vi "KelvinoxRotatorMonitor.vi"() -> ()   [LabVIEW 2019]
uses:
  Utility/Monitor Communication/Kelvinox/Kelvinox_Rotator_Cluster.ctl
  Instrument_Setup.vi
  Equipment/Mercury iXX/Public/Libraries/Auxiliary/Open/Open Auxiliary Device.vi
  Global/Global Variables/Data_Display_global.vi
  Equipment/Mercury iXX/Mercury iXX.lvlib
  Equipment/Mercury iXX/Public/Libraries/Auxiliary.lvlib
panel:
  out "Kelvinox-Rotator-Cluster":T1={"Angle (deg)"=3.4572, "Target Angle (deg)"=3.4572, "Angle SP"=0.0, "Set Angle SP"=FALSE, "Set Angle to Zero"=FALSE} {"Target Angle (deg)" format="%#.2g"; "Angle SP" format="%#.2g"; "Angle (deg)" format="%4.2g"}
  # "Kelvinox Rotator"
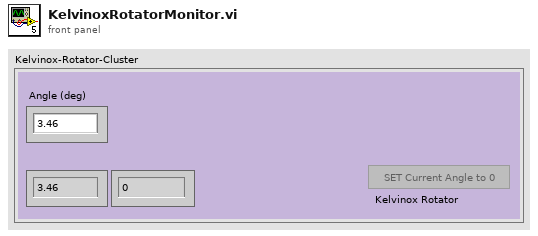
[diagram p1: front panel]
types:
  T1 = typedef "Kelvinox_Rotator_Cluster.ctl" = cluster{"Angle (deg)":dbl, "Target Angle (deg)":dbl, "Angle SP":dbl, "Set Angle SP":bool, "Set Angle to Zero":bool}
  T2 = typedef "Mercury iXX.lvlib/Mercury Reference.ctl" = cluster{"Comms":refnum<visa-resource-name>, "Device ID":string[], "Comms Layer":T3, "Command":string, "Query reference":T4}
  T3 = typedef "Mercury iXX.lvlib/Comms Transport Layer.ctl" = enum16{"Ethernet TCP/IP", "USB", "ISOBus - RS-232", "GPIB"}
  T4 = typedef "Mercury iXX.lvlib/Query Dynamic Reference.ctl" = refnum<vi>
  T5 = typedef "Kelvinox_Rotator_Control.ctl" = cluster{"Angle SP":dbl, "Set Angle SP":bool, "Set Angle to Zero":bool}
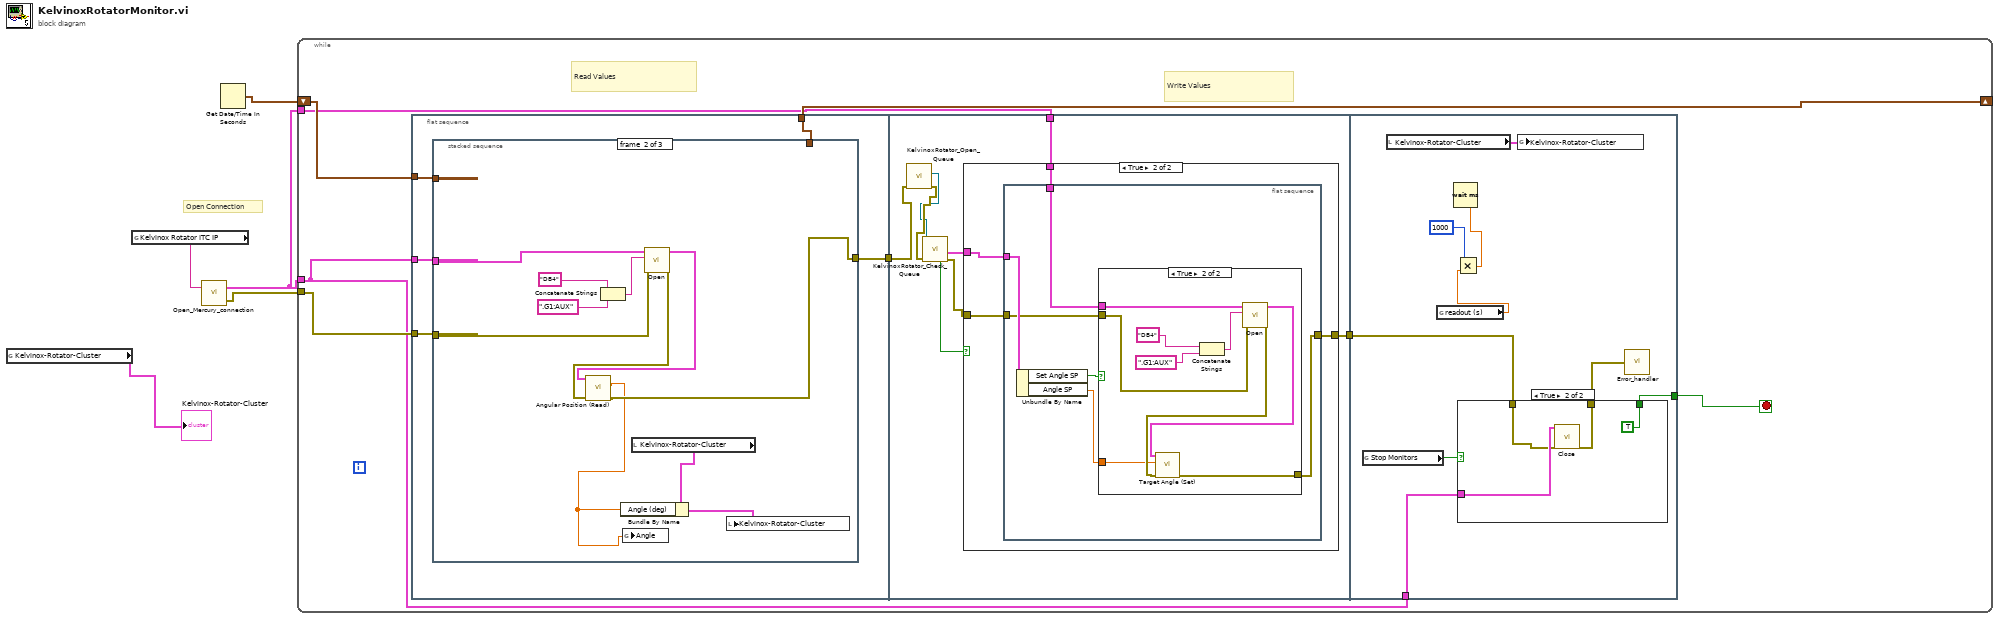
[diagram p0: block diagram]
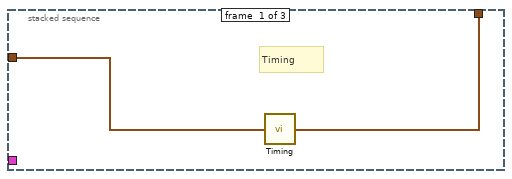
[diagram p2: hidden frame]
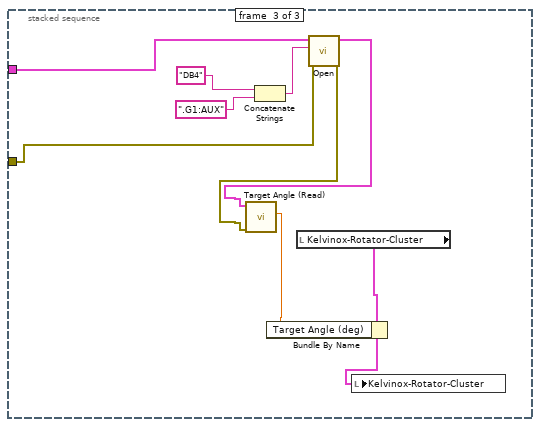
[diagram p3: hidden frame]
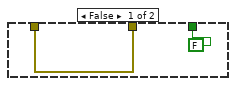
[diagram p6: hidden frame]
diagram:
  # "Open Connection"
  n1 = global read "Data_Display_global.vi" "Kelvinox-Rotator-Cluster"() -> (→"Kelvinox-Rotator-Cluster":T1)
  n2 = global read "Instrument_Setup.vi" "Kelvinox Rotator ITC IP"() -> (w5:string)
  n3 = call "Open_Mercury_connection.vi"("IP Address"=w5) -> ("error out"=w2:errorcluster, "Mercury Reference Out"=w1:T2)  [unwired: 1 in]
  n4 = Get Date/Time In Seconds() -> (seconds since 1Jan1904=w4:timestamp)
  n5 = while {
    tunnel: w1 -> [w7]
    tunnel: w2 -> [w13]
    shift-right: [w11] -> _
    shift-left: w4 -> [w12]
    tunnel: w1 -> [w9]
    stop <- w6 stop-if-true
    # "Write Values"
    # "Read Values"
    n6 = flat-sequence {
      tunnel: w13 -> [w18]
      tunnel: w7 -> [w17]
      tunnel: w12 -> [w16]
      tunnel: [w15] -> w11
      tunnel: [w14] -> w10
      tunnel: w10 -> [w47]
      tunnel: w9 -> [w49]
      tunnel: [w48] -> w8
      tunnel: w8 -> [w73]
      tunnel: w7 -> [w74]
      tunnel: [w72] -> w6
      frame #0 {
        n7 = stacked-sequence {
          tunnel: w17 -> [_ w29 w38]
          tunnel: w18 -> [_ w27 w37]
          tunnel: [_ w23 _] -> w14
          tunnel: w16 -> [w20 _ _]
          tunnel: [w19 _ _] -> w15
          frame #0 {
            # "Timing"
            n8 = call "Timing.vi"("start time (s)"=w20) -> ("last reading (s)"=w19:timestamp)
          }
          frame #1 {
            n9 = Concatenate Strings("DB4", ".G1:AUX" ("Device Identifier")) -> (w28:string)
            n10 = local read "Kelvinox-Rotator-Cluster"() -> (w22:T1)
            n11 = call-poly "Open.vi"("error in (no error)"=w27, "Device Identifier"=w28, "Mercury Reference In"=w29) -> ("error out"=w24:errorcluster, "Mercury Reference Out"=w25:T2)  [unwired: 1 in, 6 out]
            n12 = call "Angular Position (Read).vi"("error in"=w24, "Mercury Reference In"=w25) -> ("error out"=w23:errorcluster, "Position"=w21:dbl)  [unwired: 5 in, 3 out]
            n13 = Bundle By Name(cluster=w22, "Angle (deg)"=w21) -> (w26:T1)
            n14 = global write "Data_Display_global.vi" "Angle"(w21) -> ()
            n15 = local write "Kelvinox-Rotator-Cluster"(w26) -> ()
          }
          frame #2 {
            n16 = Concatenate Strings("DB4", ".G1:AUX" ("Device Identifier")) -> (w41:string)
            n17 = local read "Kelvinox-Rotator-Cluster"() -> (w32:T1)
            n18 = call-poly "Open.vi"("error in (no error)"=w37, "Device Identifier"=w41, "Mercury Reference In"=w38) -> ("error out"=w35:errorcluster, "Mercury Reference Out"=w36:T2)  [unwired: 1 in, 6 out]
            n19 = call "Target Angle (Read).vi"("error in"=w35, "Mercury Reference In"=w36) -> ("Position"=w34:dbl)  [unwired: 5 in, 4 out]
            n20 = Bundle By Name(cluster=w32, "Target Angle (deg)"=w34) -> (w33:T1)
            n21 = local write "Kelvinox-Rotator-Cluster"(w33) -> ()
          }
        }
      }
      frame #1 {
        n22 = call "KelvinoxRotator_Open_Queue.vi"("error in (no error)"=w47) -> ("error out"=w43:errorcluster, "queue out"=w42:refnum<queue>)  [unwired: 9 in]
        n23 = call "KelvinoxRotator_Check_Queue.vi"("error in (no error)"=w43, "queue"=w42) -> ("error out"=w44:errorcluster, "Kelvinox-Rotator-Control"=w46:T5, "New Entries?"=w45:bool)  [unwired: 6 in]
        n24 = case shown="True" w45 {
          tunnel: w46 -> [_ w54]
          tunnel: w49 -> [_ w53]
          tunnel: w44 -> [w50 w52]
          tunnel: [w50 w51] -> w48
          frame False {
          }
          frame True {
            n25 = flat-sequence {
              tunnel: w54 -> [w60]
              tunnel: w53 -> [w59]
              tunnel: w52 -> [w57]
              tunnel: [w55] -> w51
              frame #0 {
                n26 = Unbundle By Name(w60) -> ("Set Angle SP"=w58:bool, "Angle SP"=w56:dbl)
                n27 = case shown="True" w58 {
                  tunnel: w59 -> [_ w67]
                  tunnel: w57 -> [w61 w65]
                  tunnel: w56 -> [_ w63]
                  tunnel: [w61 w62] -> w55
                  frame False {
                  }
                  frame True {
                    n28 = Concatenate Strings("DB4", ".G1:AUX" ("Device Identifier")) -> (w70:string)
                    n29 = call-poly "Open.vi"("error in (no error)"=w65, "Device Identifier"=w70, "Mercury Reference In"=w67) -> ("error out"=w64:errorcluster, "Mercury Reference Out"=w66:T2)  [unwired: 1 in, 6 out]
                    n30 = call "Target Angle (Set).vi"("error in"=w64, "Position"=w63, "Mercury Reference In"=w66) -> ("error out"=w62:errorcluster)  [unwired: 5 in, 3 out]
                  }
                }
              }
            }
          }
        }
      }
      frame #2 {
        n31 = global read "Data_Display_global.vi" "Stop Monitors"() -> (w75:bool)
        n32 = local read "Kelvinox-Rotator-Cluster"() -> (w79:T1)
        n33 = global read "Instrument_Setup.vi" "readout (s)"() -> (w77:dbl)
        n34 = Multiply(x=1000, y=w77) -> (x*y=w78:dbl)
        n35 = Wait (ms)(milliseconds to wait=w78) -> ()  [unwired: 1 out]
        n36 = case shown="True" w75 {
          tunnel: w74 -> [_ w85]
          tunnel: [w80 w82] -> w71
          tunnel: [FALSE TRUE] -> w72
          tunnel: w73 -> [w80 w83]
          frame False {
          }
          frame True {
            n37 = call "Close.vi"("error in (no error)"=w83, "Mercury Reference"=w85) -> ("error out"=w82:errorcluster)  [unwired: 9 in]
          }
        }
        n38 = global write "Data_Display_global.vi" "Kelvinox-Rotator-Cluster"(w79) -> ()
        n39 = call "Error_handler.vi"("error constant"=w71) -> ()
      }
    }
  }
